vi "LocalVariable_declaration.vi"() -> ()   [LabVIEW 2019]
panel:
  out "x^2":dbl
  out "result":dbl
  in  "Numeric 3":dbl=10.0
  in  "Numeric 2":dbl=8.0
  in  "Numeric 1":dbl=4.0
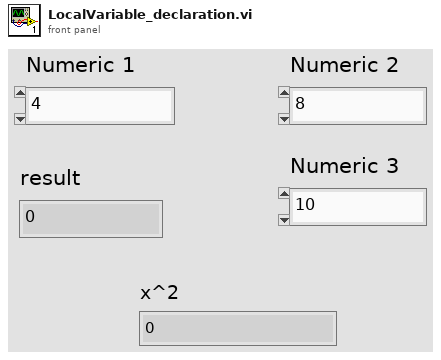
[diagram p1: front panel]
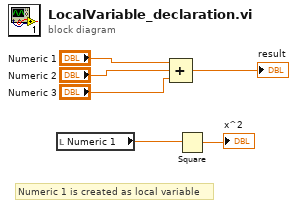
[diagram p0: block diagram]
diagram:
  # "Numeric 1 is created as local variable"
  n1 = local read "Numeric 1"() -> (w2:dbl)
  n2 = Compound Arithmetic op=ADD("Numeric 1", "Numeric 2", "Numeric 3") -> (→"result":dbl)
  n3 = Square(x=w2) -> (x^2=→"x^2":dbl)
